vi "IntakeGlobal.vi"() -> ()   [LabVIEW 2020]
panel:
  out "turntableDemand":dbl
  out "intakeLowerDemand":dbl
  out "intakeUpperDemand":dbl
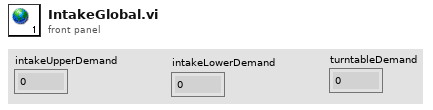
[diagram p1: front panel]
diagram:
